vi "MulticolumnListbox - clean.vi"(7 "MulticolumnListbox":refnum<vi>) -> ()   [LabVIEW 2017, in "util.lvlib"]
uses:
  util.lvlib
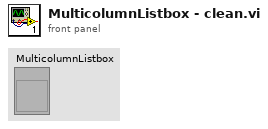
[diagram p1: front panel]
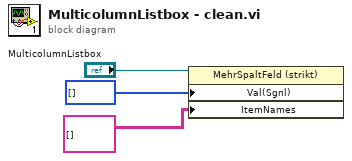
[diagram p0: block diagram]
diagram:
  n1 = property class="MehrSpaltFeld (strikt)"(reference="MulticolumnListbox", "Val(Sgnl)"=i32[] [] ("Wert (signalisierend)"), "ItemNames"=string[][] [] ("Objektnamen")) -> ()  [unwired: 1 in, 2 out]
